vi "lab3_task3.vi"() -> ()   [LabVIEW 2021]
uses:
  <vilib>/Utility/file.llb/Write Delimited Spreadsheet (DBL).vi
  <vilib>/express/express analysis/Spectral/Block/exnSpectralBlock spectral measurements PSD poly.vi
  <vilib>/express/express analysis/Spectral/Block/exnSpectralBlock spectral measurements PSD DDT.vi
  <vilib>/express/express analysis/Spectral/XNode/ExpressSpectralMeasurementsBlockNode.xnode
  <vilib>/Analysis/NI_AALPro.lvlib
panel:
  out "Waveform Graph":dynamicdata(graph)
  in  "# bins":i32
  out "Histogram Graph":T1(graph)
  in  "file path (dialog if empty)":path
  out "rms":dbl
  out "peak to peak":dbl
  out "mean":dbl
  out "data":dynamicdata(graph)
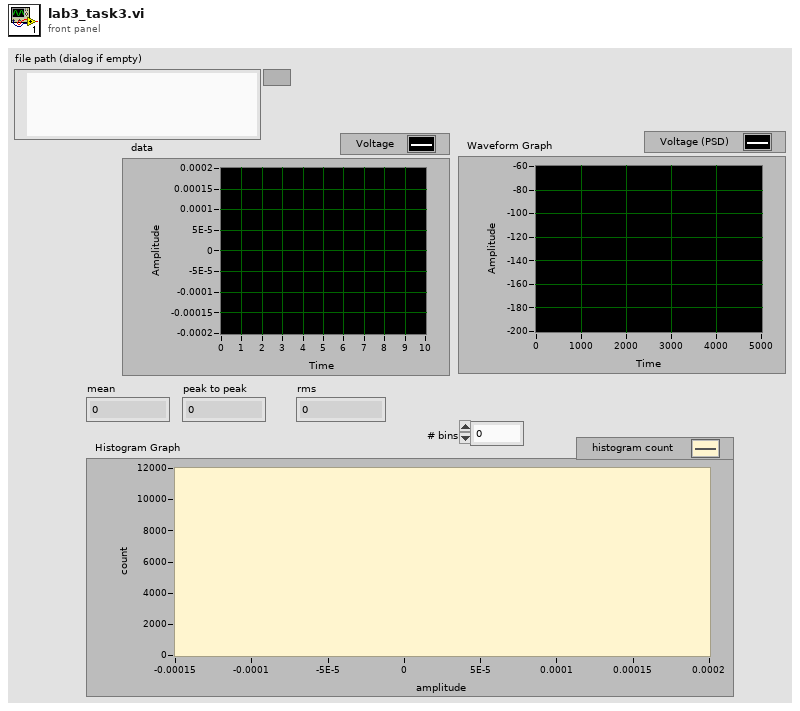
[diagram p1: front panel]
types:
  T1 = cluster{"X Values":dbl[], "Histogram: h(x)":i32[]}
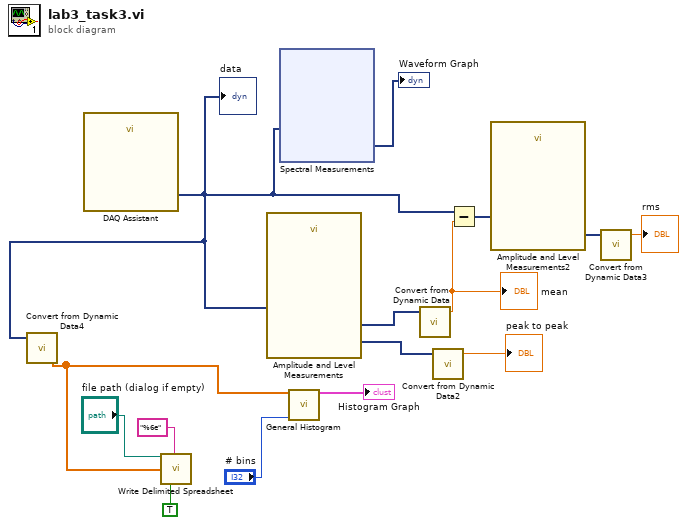
[diagram p0: block diagram]
diagram:
  n1 = call "DAQ Assistant"() -> ("data"=w2:dynamicdata)  [unwired: 17 in, 2 out]
  "data" <- w2
  n2 = call "Convert from Dynamic Data4"("Dynamic Data Type"=w2) -> ("Array"=w3:dbl[])  [unwired: 3 in]
  n3 = call-poly <vilib>:"Write Delimited Spreadsheet.vi"("file path (dialog if empty)"="file path (dialog if empty)", "format (%.3f)"="%6e", "1D data"=w3, "transpose? (no:F)"=TRUE) -> ()  [unwired: 10 in, 2 out]
  n4 = call "Amplitude and Level Measurements"("Signals"=w2) -> ("Mean (DC)"=w15:dynamicdata, "Peak to Peak"=w14:dynamicdata)  [unwired: 12 in, 1 out]
  n5 = xnode "Spectral Measurements"("Signals"=w2) -> ("PSD"=→"Waveform Graph":dynamicdata)  [unwired: 1 in, 1 out]
  n6 = call <vilib>:"General Histogram.vi"("X"=w3, "# bins"="# bins") -> ("Histogram Graph"=→"Histogram Graph":T1)  [unwired: 9 in, 4 out]
  n7 = call "Convert from Dynamic Data"("Dynamic Data Type"=w15) -> ("Scalar"=w12:dbl)  [unwired: 3 in]
  "mean" <- w12
  n8 = call "Convert from Dynamic Data2"("Dynamic Data Type"=w14) -> ("Scalar"=→"peak to peak":dbl)  [unwired: 3 in]
  n9 = Subtract(x=w2, y=w12) -> (x-y=w11:dynamicdata)
  n10 = call "Amplitude and Level Measurements2"("Signals"=w11) -> ("RMS"=w10:dynamicdata)  [unwired: 13 in, 1 out]
  n11 = call "Convert from Dynamic Data3"("Dynamic Data Type"=w10) -> ("Scalar"=→"rms":dbl)  [unwired: 3 in]
